vi "Write delta pres.vi"(10 "delta pres":dbl, 11 "ValveModbus in":refnum<class "NeedleValve.lvclass">) -> (3 "ValveModbus out":refnum<class "NeedleValve.lvclass">)   [LabVIEW 2019]
uses:
  NeedleValve.lvclass
  D:/GIT H4000/H4000/src/Device_class/Device.lvclass
  D:/GIT H4000/H4000/src/Proccess_class/Proccess.lvclass
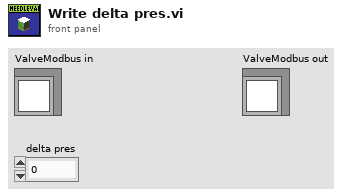
[diagram p1: front panel]
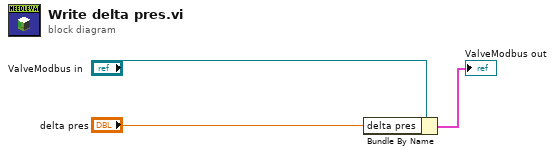
[diagram p0: block diagram]
diagram:
  n1 = Bundle By Name(cluster="ValveModbus in", "delta pres"="delta pres") -> (→"ValveModbus out":cluster{})
